vi "Do.vi"(8 "error in (no error)":errorcluster, 10 "Actor in":refnum<class "Actor.lvclass">, 11 "Send Log Message MSG":refnum<class "Send Log Message MSG.lvclass">) -> (0 "error out":errorcluster, 2 "Actor out":refnum<class "Actor.lvclass">)   [LabVIEW 2014, in "Controller.lvlib" / "Send Log Message MSG.lvclass"]
doc: "(<B>Filename</B>: Actor Framework.lvlib:Message.lvclass:Do.vi)\n\nDefines what a message does when it is received by an actor. Generally, a message instructs an actor to invoke one of its methods. By default, this method does nothing. A child class must override it to define behavior. Create a child class by using the Actor Framework Message Maker dialog box."
uses:
  Send Log Message MSG.lvclass
  <vilib>/ActorFramework/Actor/Actor.lvclass
  Send Log Message MSG.lvclass/Send Log Message MSG.ctl
  Controller.lvclass
  SuperActor/SuperActor.lvclass/SuperActor.ctl
  SuperActor/Read Log Session.vi
  <userlib>/_Session Fwk/Session - Root.lvclass
  reusable/Session APIs/Session Log/System Log.lvclass
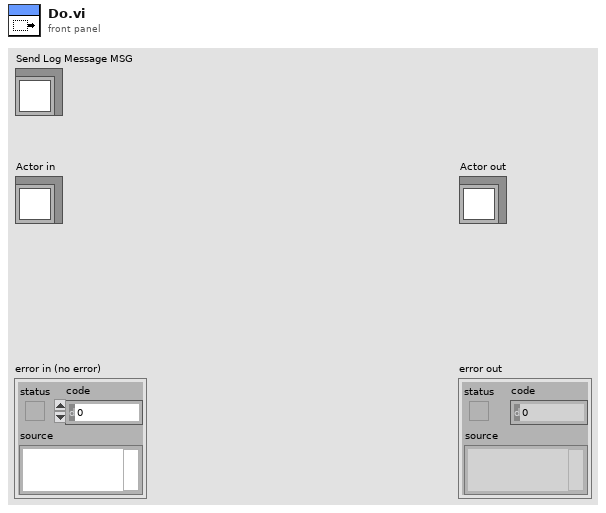
[diagram p1: front panel]
types:
  T1 = typedef "Session - Root.lvclass/Session Handle.ctl" = refnum<data-value>
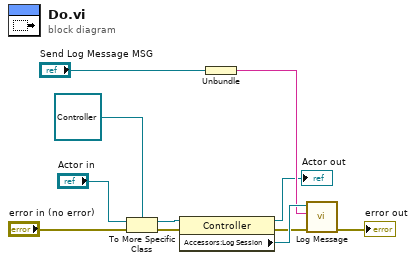
[diagram p0: block diagram]
diagram:
  n1 = To More Specific Class(target class=refnum<class "Controller.lvclass"> refnum ("Controller:Controller"), reference="Actor in", error in="error in (no error)") -> (specific class reference=w8:refnum<class "Controller.lvclass">, error out=w7:errorcluster)
  n2 = property class="Controller"(reference=w8, error in=w7) -> (reference out=→"Actor out":refnum<class "Controller.lvclass">, error out=w4:errorcluster, "Accessors:Log Session"=w6:T1)
  n3 = Unbundle("Send Log Message MSG") -> (w5:string)
  n4 = call "Log Message.vi"("error in"=w4, "MSG In"=w5, "session in"=w6) -> ("error out"=→"error out":errorcluster)  [unwired: 7 in, 1 out]
